vi "fg_class.vi"(7 "fg_command":T1=enum."read", 8 "error in (no error)":errorcluster, 11 "class in":refnum<class "v1.lvclass">) -> (0 "error out":errorcluster, 3 "class out":refnum<class "v1.lvclass">)   [LabVIEW 2015, in "lv-dialog.lvlib" / "v1.lvlib"]
uses:
  v1.lvlib
  public/class/v1.lvclass
  _controls/fg_command.ctl
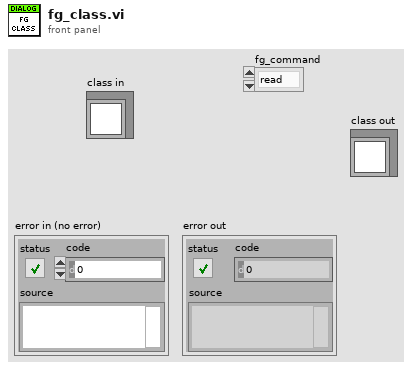
[diagram p1: front panel]
types:
  T1 = typedef "lv-dialog.lvlib/v1.lvlib/fg_command.ctl" = enum16{"null", "initialize", "read", "write", "shutdown"}
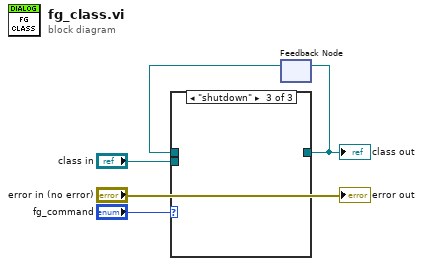
[diagram p0: block diagram]
diagram:
  n1 = feedback #1() -> (w2:refnum<class "v1.lvclass">)  [unwired: 1 in]
  n2 = case shown="\"shutdown\"" "fg_command" {
    tunnel: w2 -> [_ w7 _]
    tunnel: [w6 w7 _] -> w3
    tunnel: "class in" -> [w6 _ _]
    frame "initialize", "write" {
    }
    frame Default {
    }
    frame "shutdown" {
    }
  }
  "class out" <- w3
  n3 = feedback-in #1(w3) -> ()
  "error out" <- "error in (no error)"
